vi "sensor_nivel_linx2.vi"() -> ()   [LabVIEW 2018]
doc: "This example demonstrates how to read N channels of analog input from a LINX device."
uses:
  <vilib>/MakerHub/LINX/Public/Peripherals/Analog/Analog Read 1 Chan.vi
  <vilib>/MakerHub/LINX/Public/Peripherals/Analog/Analog Read N Chans.vi
  <vilib>/MakerHub/LINX/Private/Local IO/LinxAnalogRead.vi
  <vilib>/MakerHub/LINX/Public/Utilities/Check Channel.vi
  <vilib>/MakerHub/LINX/Public/Utilities/Open Serial.vi
  <vilib>/MakerHub/LINX/Private/Utilties/Generate Error.vi
  <vilib>/MakerHub/LINX/LMH-LINX.lvlib
panel:
  out "?":cluster{dbl, dbl}(graph)
  out "CAIXAS":dbl format="%_3g"
  out "CISTERNAS":dbl format="%_3g"
  in  "?":dbl
  out "CISTERNAS":bool
  in  "?":dbl
  out "CAIXAS":bool
  in  "Intervalo de leituras":u32
  out "Caixa 2":dbl(slide) scale=0.0..30.0
  out "Cisterna 2":dbl(slide) scale=0.0..30.0
  in  "Stop Button":bool
  in  "?":refnum<visa-resource-name>
  out "Cisterna 1":dbl(slide) scale=0.0..30.0
  out "Caixa 1":dbl(slide) scale=0.0..30.0
  # "CONTROLE DE NÍVEL DE ÁGUA"
  # "VOLUME x 1000L"
  # "ALARMES"
  # "AJUSTE NÍVEL BAIXO"
  # "AJUSTE NÍVEL BAIXO"
  # "Controles"
  # "Porta Serial"
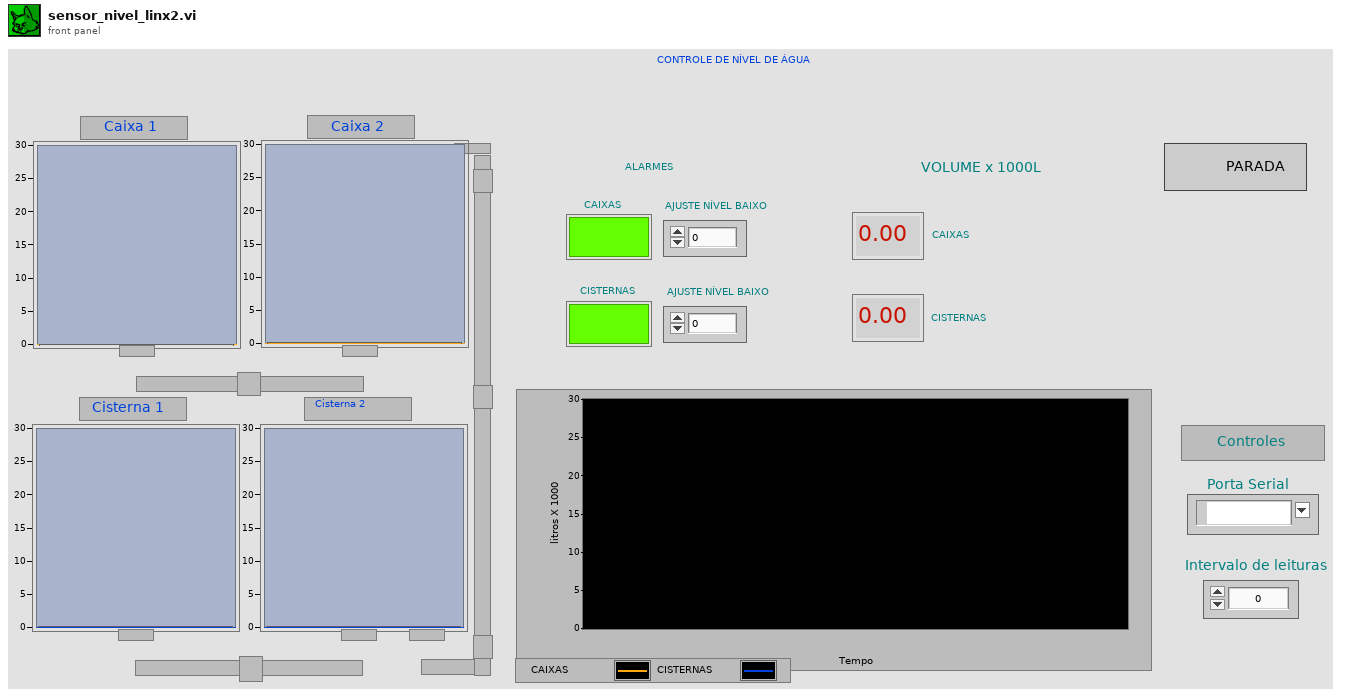
[diagram p1: front panel]
types:
  T1 = typedef "LMH-LINX.lvlib/LINX Ref.ctl" = cluster{"IO":T2, "Interface":T3, "LINX Device Config":T4}
  T2 = typedef "LMH-LINX.lvlib/Platform.ctl" = enum16{"Remote", "Local"}
  T3 = typedef "LMH-LINX.lvlib/Interface.ctl" = enum16{"Serial", "TCP"}
  T4 = typedef "LMH-LINX.lvlib/Device.lvlib/LINX Device Config.ctl" = cluster{"Interface":T3, "COM Port":refnum<visa-resource-name>, "TCP Configuration":T5, "Device Family":u8, "Device ID":u8, "Device Name":string, "TCP Ref":refnum<k5>, "Channels":T6}
  T5 = typedef "LMH-LINX.lvlib/Device.lvlib/TCP Config.ctl" = cluster{"IP Address":string, "Port":u16}
  T6 = typedef "LMH-LINX.lvlib/Channels.ctl" = cluster{"DI":u8[], "DO":u8[], "AI":u8[], "AO":u8[], "PWM":u8[], "QE":u8[], "UART":u8[], "I2C 2":u8[], "SPI":u8[], "CAN":u8[], "Servo":u8[], "AI Ref (V)":dbl, "AI Resolution (Bits)":u8, "AO Ref (V)":dbl, "AO Resolution (Bits)":u8}
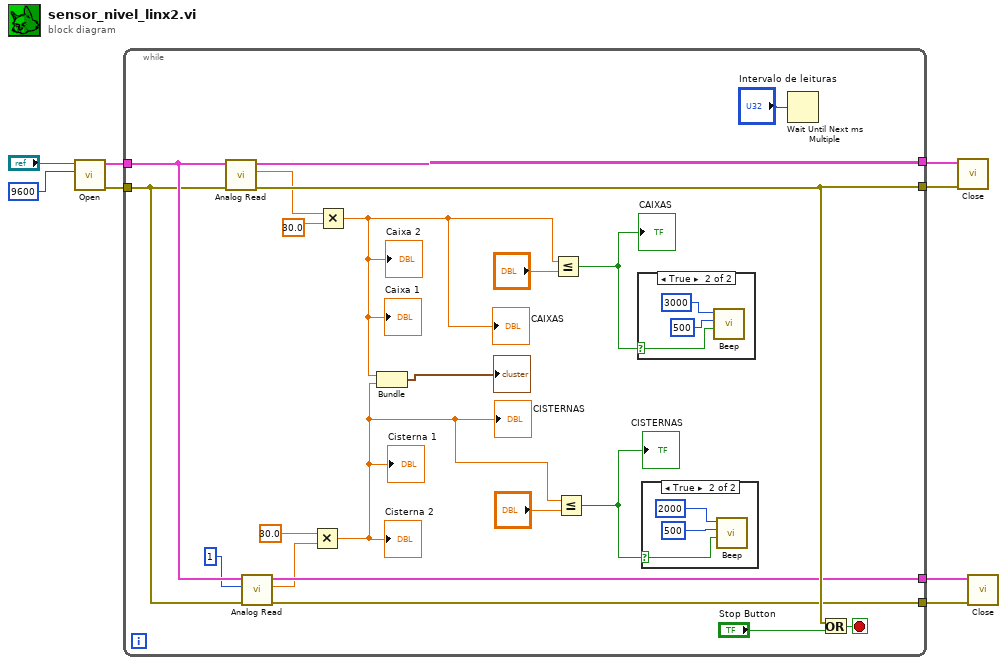
[diagram p0: block diagram]
diagram:
  n1 = call-poly <vilib>:"Open.vi"("Baud Rate Override"=u32 9600, "Serial Port"="?") -> ("Error Out"=w5:errorcluster, "LINX Resource"=w8:T1)  [unwired: 7 in, 1 out]
  n2 = while {
    tunnel: w8 -> [w26]
    tunnel: [w28] -> w6
    tunnel: w5 -> [w25]
    tunnel: [w27] -> w4
    tunnel: [w24] -> w3
    tunnel: [w23] -> w2
    stop <- w29 stop-if-true
    n3 = call-poly <vilib>:"Analog Read.vi"("Error In"=w25, "LINX Resource"=w26) -> ("Error Out"=w28:errorcluster, "Voltage"=w21:dbl, "LINX Resource"=w27:T1)  [unwired: 6 in, 1 out]
    n4 = call-poly <vilib>:"Analog Read.vi"("Error In"=w25, "Analog Channel"=u8 1, "LINX Resource"=w26) -> ("Error Out"=w23:errorcluster, "Voltage"=w19:dbl, "LINX Resource"=w24:T1)  [unwired: 5 in, 1 out]
    n5 = Multiply(x=30.0, y=w19) -> (x*y=w14:dbl)
    "Cisterna 1" <- w14
    "Cisterna 2" <- w14
    "CISTERNAS" <- w14
    n6 = Multiply(x=w21, y=30.0) -> (x*y=w11:dbl)
    "Caixa 1" <- w11
    "Caixa 2" <- w11
    "CAIXAS" <- w11
    n7 = Bundle(w11, w14) -> (→"?":cluster{dbl, dbl})  [unwired: 1 in]
    n8 = Less Or Equal?(x=w11, y="?") -> (x <= y?=w12:bool)
    "CAIXAS" <- w12
    n9 = Less Or Equal?(x=w14, y="?") -> (x <= y?=w15:bool)
    "CISTERNAS" <- w15
    n10 = case shown="True" w12 {
      selector: w12 -> [_ w30]
      frame False {
      }
      frame True {
        n11 = call <vilib>:"Beep.vi"("use system alert? (T)"=w30, "duration (msec)"=u32 500, "frequency (Hz)"=u32 3000) -> ()  [unwired: 9 in]
      }
    }
    n12 = case shown="True" w15 {
      selector: w15 -> [_ w33]
      frame False {
      }
      frame True {
        n13 = call <vilib>:"Beep.vi"("use system alert? (T)"=w33, "duration (msec)"=u32 500, "frequency (Hz)"=u32 2000) -> ()  [unwired: 9 in]
      }
    }
    n14 = Wait Until Next ms Multiple(millisecond multiple="Intervalo de leituras") -> ()  [unwired: 1 out]
    n15 = Or(x=w28, y="Stop Button") -> (x .or. y?=w29:bool)
  }
  n16 = call <vilib>:"Close.vi"("Error In"=w6, "LINX Resource"=w4) -> ()  [unwired: 9 in, 1 out]
  n17 = call <vilib>:"Close.vi"("Error In"=w2, "LINX Resource"=w3) -> ()  [unwired: 9 in, 1 out]
